vi "SPOL_temps.vi"() -> ()   [LabVIEW 2009]
uses:
  <vilib>/Utility/file.llb/Write To Spreadsheet File (DBL).vi
  <vilib>/Utility/file.llb/Write To Spreadsheet File (string).vi
panel:
  out "Temperatures":T1(graph)
  out "Next Sample":dbl format="%.3g"
  in  "loop time(ms)":u32=10
  out "Samples":i32
  in  "stop":bool
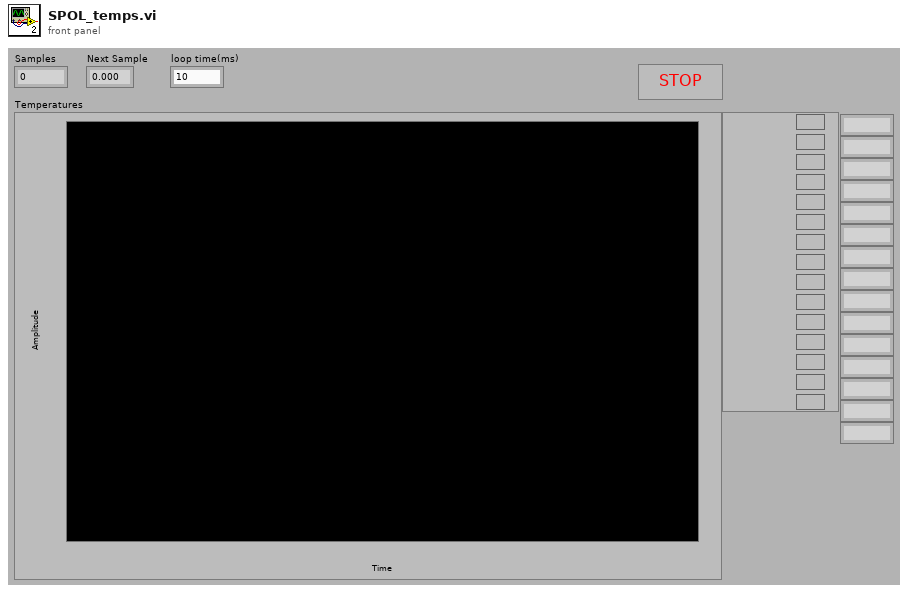
[diagram p1: front panel]
types:
  T1 = cluster{"[0]":dbl, "[1]":dbl, "[2]":dbl, "[3]":dbl, "[4]":dbl, "[5]":dbl, "[6]":dbl, "[7]":dbl, "[8]":dbl, "[9]":dbl, "[10]":dbl, "[11]":dbl, "[12]":dbl, "[13]":dbl, "[14]":dbl}
  T2 = cluster{"[0]":dbl, "[1]":dbl, "[2]":dbl, "[3]":dbl, "[4]":dbl, "[5]":dbl, "[6]":dbl, "[7]":dbl, "[8]":dbl, "[9]":dbl, "[10]":dbl, "[11]":dbl, "[12]":dbl, "[13]":dbl, "[14]":dbl}[]
  T3 = typedef "LVDateTimeRec.ctl" = cluster{"fractional second":dbl, "second":i32, "minute":i32, "hour":i32, "day of month":i32, "month":i32, "year":i32, "day of week":i32, "day of year":i32, "DST":i32}
  T4 = cluster{"Temperatures[0]":dbl, "Temperatures[1]":dbl, "Temperatures[2]":dbl, "Temperatures[3]":dbl, "Temperatures[4]":dbl, "Temperatures[5]":dbl, "Temperatures[6]":dbl, "Temperatures[7]":dbl, "Temperatures[8]":dbl, "Temperatures[9]":dbl, "Temperatures[10]":dbl, "Temperatures[11]":dbl, "Temperatures[12]":dbl, "Temperatures[13]":dbl, "Temperatures[14]":dbl}
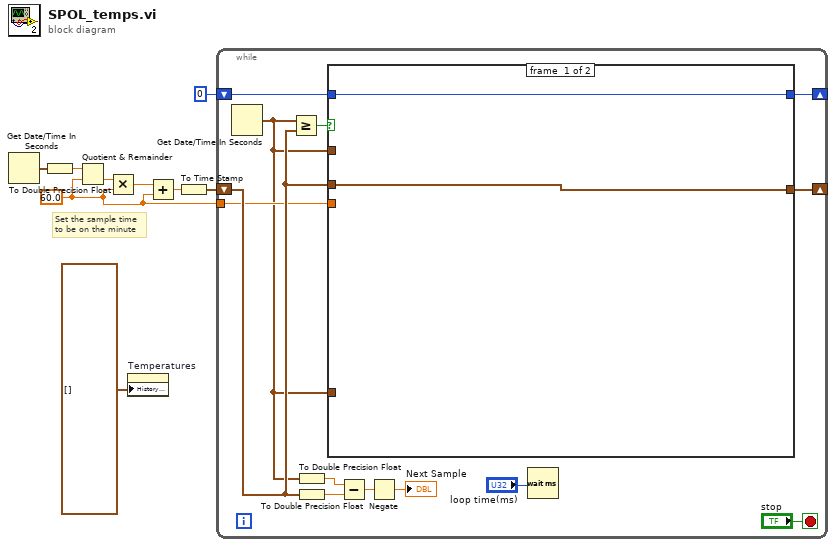
[diagram p0: block diagram]
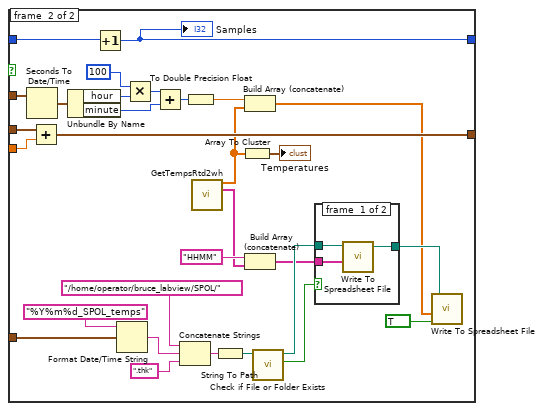
[diagram p2: hidden frame]
diagram:
  w3 = 60.0 ("y")
  # "Set the sample time\nto be on the minute"
  n1 = Get Date/Time In Seconds() -> (seconds since 1Jan1904=w2:timestamp)
  n2 = To Double Precision Float(number=w2) -> (double precision float=w9:dbl)
  n3 = Quotient & Remainder(x=w9, y=w3) -> (floor(x/y)=w7:dbl)  [unwired: 1 out]
  n4 = Multiply(x=w7, y=w3) -> (x*y=w8:dbl)
  n5 = property on="Temperatures" class="WFChart (strict)"("History Data"=T2 []) -> ()  [unwired: 2 in, 2 out]
  n6 = Add(x=w8, y=w3) -> (x+y=w6:dbl)
  n7 = To Time Stamp(1:w6) -> (0:w4:timestamp)
  n8 = while {
    tunnel: w3 -> [w13]
    shift-right: [w22] -> _
    shift-left: w4 -> [w18]
    shift-right: [w20] -> _
    shift-left: 0 -> [w21]
    stop <- "stop" stop-if-true
    n9 = Get Date/Time In Seconds() -> (seconds since 1Jan1904=w10:timestamp)
    n10 = Greater Or Equal?(x=w10, y=w18) -> (x >= y?=w19:bool)
    n11 = To Double Precision Float(number=w10) -> (double precision float=w17:dbl)
    n12 = To Double Precision Float(number=w18) -> (double precision float=w16:dbl)
    n13 = case shown="True" w19 {
      tunnel: w18 -> [w24 w51]
      tunnel: [w24 w54] -> w22
      tunnel: w21 -> [w23 w53]
      tunnel: [w23 w52] -> w20
      tunnel: w10 -> [_ w50]
      tunnel: w13 -> [_ w49]
      tunnel: w10 -> [_ w25]
      frame #0 {
      }
      frame #1 {
        n14 = Seconds To Date/Time(time stamp (now)=w50) -> (date time rec=w44:T3)  [unwired: 1 in]
        n15 = Add(x=w51, y=w49) -> (x+y=w54:timestamp)
        n16 = Unbundle By Name(w44) -> ("hour"=w43:i32, "minute"=w40:i32)
        n17 = Increment(x=w53) -> (x+1=w52:i32)
        "Samples" <- w52
        n18 = Format Date/Time String(time format string (%c)="%Y%m%d_SPOL_temps", seconds (now)=w25) -> (date/time string=w31:string)  [unwired: 1 in]
        n19 = Multiply(x=100, y=w43) -> (x*y=w41:i32)
        n20 = Add(x=w41, y=w40) -> (x+y=w36:i32)
        n21 = Concatenate Strings("/home/operator/bruce_labview/SPOL/", w31, ".thk" ("string")) -> (w33:string)
        n22 = To Double Precision Float(number=w36) -> (double precision float=w35:dbl)
        n23 = call "GetTempsRtd2wh.vi"() -> ("Temperatures"=w28:dbl[], "Variables"=w38:string[])  [unwired: 12 in, 2 out]
        n24 = String To Path(string=w33) -> (path=w26:path)
        n25 = Array To Cluster(array=w28) -> (cluster=→"Temperatures":T4)
        n26 = Build Array (concatenate)(w35, w28) -> (w34:dbl[])
        n27 = Build Array (concatenate)("HHMM", w38) -> (w37:string[])
        n28 = call <vilib>:"Check if File or Folder Exists.vi"("path"=w26) -> ("file or folder exists?"=w46:bool, "dup path"=w47:path)  [unwired: 8 in, 1 out]
        n29 = case shown="False" w46 {
          tunnel: w47 -> [w57 w58]
          tunnel: w37 -> [w56 _]
          tunnel: [w55 w58] -> w45
          frame #0 {
            n30 = call-poly <vilib>:"Write To Spreadsheet File.vi"("1D data"=w56, "file path (dialog if empty)"=w57) -> ("new file path (Not A Path if cancelled)"=w55:path)  [unwired: 6 in]
          }
          frame #1 {
          }
        }
        n31 = call-poly <vilib>:"Write To Spreadsheet File.vi"("append to file? (new file:F)"=TRUE, "1D data"=w34, "file path (dialog if empty)"=w45) -> ()  [unwired: 5 in, 1 out]
      }
    }
    n32 = Subtract(x=w17, y=w16) -> (x-y=w15:dbl)
    n33 = Negate(x=w15) -> (-x=→"Next Sample":dbl)
    n34 = Wait (ms)(milliseconds to wait="loop time(ms)") -> ()  [unwired: 1 out]
  }
